vi "DriveDataAQ.vi"(8 "Reset?":bool) -> (2 "Throttle Out":dbl)   [LabVIEW 2015]
uses:
  navX-MXP Library/COMMON/TypeDefs/Data TypeDefs/navX Vector Data.ctl
  navX-MXP Library/navX-MXP IMU.lvlib
panel:
  out "Raw Output Z":dbl[][](array[numeric])
  out "Raw Output Y":dbl[][](array[numeric])
  out "Valid?":bool
  out "Raw Output X":dbl[][](array[numeric])
  out "Linear Acceleration":T1
  in  "Set Throttle":dbl
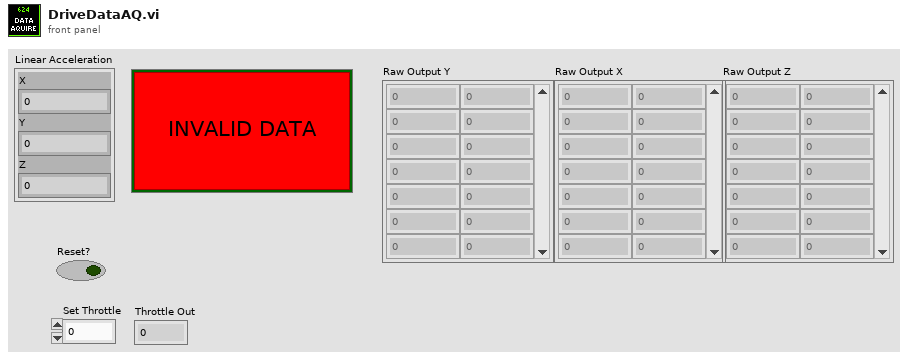
[diagram p1: front panel]
types:
  T1 = typedef "navX-MXP IMU.lvlib/navX Vector Data.ctl" = cluster{"X":dbl, "Y":dbl, "Z":dbl}
  T2 = typedef "navX-MXP IMU.lvlib/navX Device TypeDef.ctl" = cluster{"navX Interface Protocol":T3, "navX Interface Protocol TypeDefs":cluster{"SPIDevRef":T4, "I2CDevRef":T6}, "navX System Information":cluster{"Board Information":T8, "Status":T9, "Offsets":T13}, "navX Common Information":cluster{"Update Rate (4Hz-60Hz)":T14, "refnum name":string, "error":errorcluster}}
  T3 = typedef "navX-MXP IMU.lvlib/navX Interface Protocol.ctl" = enum16{"SPI", "I2C"}
  T4 = typedef "WPI_SPIDevRef.ctl" = cluster{"DevStatus":errorcluster, "Handle":i32, "SPI Bus":T5}
  T5 = typedef "spi_bus.ctl" = enum16{"SPI On-Board, CS0", "SPI On-Board, CS1", "SPI On-Board, CS2", "SPI On-Board, CS3", "SPI MXP", "Invalid"}
  T6 = typedef "WPI_I2CDevRef.ctl" = cluster{"DevStatus":errorcluster, "Device Address":u8, "Handle":i32, "I2C Bus":T7}
  T7 = typedef "i2c_bus.ctl" = enum16{"I2C On-Board", "I2C MXP", "Invalid"}
  T8 = typedef "navX-MXP IMU.lvlib/navX Board Information.ctl" = cluster{"WhoAmI (50 | 0x32)":u8, "Board Revision":u8, "Firmware Major Version":u8, "Firmware Minor Version":u8}
  T9 = typedef "navX-MXP IMU.lvlib/navX Status Data.ctl" = cluster{"Update Rate Hz":u8, "Accelerometer Full-Scale Range":u8, "Gyro Full-Scale Range":u16, "NAVX_OP_STATUS":T10, "NAVX_CAL_STATUS":T11, "NAVX_SELFTEST_STATUS":u8, "NAVX_SENSOR_STATUS":T12}
  T10 = typedef "navX-MXP IMU.lvlib/navX NAVX_OP_STATUS.ctl" = u8
  T11 = typedef "navX-MXP IMU.lvlib/navX NAVX_CAL_STATUS.ctl" = u8
  T12 = typedef "navX-MXP IMU.lvlib/navX NAVX_SENSOR_STATUS.ctl" = cluster{"MOVING":bool, "YAW_STABLE":bool, "MAG_DISTURBANCE":bool, "ALTITUDE_VALID":bool, "SEALEVEL_PRESS_SET":bool, "FUSED_HEADING_VALID":bool}
  T13 = typedef "navX-MXP IMU.lvlib/navX Offsets Data.ctl" = cluster{"Yaw":dbl, "Quat W":dbl, "Quat X":dbl, "Quat Y":dbl, "Quat Z":dbl}
  T14 = typedef "navX-MXP IMU.lvlib/navX Update Rate.ctl" = u8
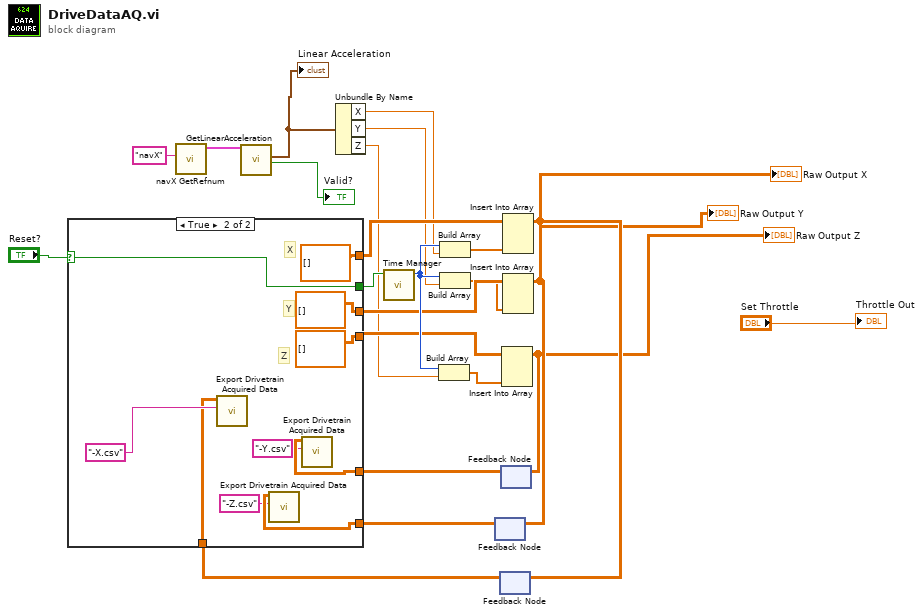
[diagram p0: block diagram]
diagram:
  n1 = call "navX GetRefnum.vi"("refnum name"="navX") -> ("navX Device TypeDef"=w18:T2)  [unwired: 9 in, 1 out]
  n2 = call "GetLinearAcceleration.vi"("navX Device TypeDef"=w18) -> ("Valid?"=→"Valid?":bool, "Linear Acceleration"=w8:T1)  [unwired: 8 in, 1 out]
  "Linear Acceleration" <- w8
  n3 = Unbundle By Name(w8) -> ("X"=w2:dbl, "Y"=w1:dbl, "Z"=w3:dbl)
  n4 = feedback #1() -> (w11:dbl[][])  [unwired: 1 in]
  n5 = feedback #2() -> (w22:dbl[][])  [unwired: 1 in]
  n6 = feedback #3() -> (w10:dbl[][])  [unwired: 1 in]
  n7 = case shown="True" "Reset?" {
    selector: "Reset?" -> [w26 w36]
    tunnel: [w27 dbl[][] []] -> w23
    tunnel: w22 -> [w27 w32]
    tunnel: [w26 w36] -> w20
    tunnel: [w25 dbl[][] []] -> w15
    tunnel: [w24 dbl[][] []] -> w14
    tunnel: w11 -> [w25 w29]
    tunnel: w10 -> [w24 w31]
    frame False {
    }
    frame True {
      # "Z"
      # "Y"
      # "X"
      n8 = call "Export Drivetrain Acquired Data.vi"("string"="-X.csv", "Array"=w32) -> ()  [unwired: 10 in]
      n9 = call "Export Drivetrain Acquired Data.vi"("string"="-Z.csv", "Array"=w29) -> ()  [unwired: 10 in]
      n10 = call "Export Drivetrain Acquired Data.vi"("string"="-Y.csv", "Array"=w31) -> ()  [unwired: 10 in]
    }
  }
  n11 = call "Time Manager.vi"("Reset?"=w20) -> ("Elapsed Time"=w16:u32)  [unwired: 10 in]
  n12 = Build Array(w16, w3) -> (w13:dbl[])
  n13 = Build Array(w16, w2) -> (w19:dbl[])
  n14 = Build Array(w16, w1) -> (w12:dbl[])
  n15 = Insert Into Array(array=w14, new element=w13) -> (w4:dbl[][])  [unwired: 2 in]
  "Raw Output Z" <- w4
  n16 = feedback-in #3(w4) -> ()
  n17 = Insert Into Array(array=w23, new element=w19) -> (w6:dbl[][])  [unwired: 2 in]
  "Raw Output X" <- w6
  n18 = feedback-in #2(w6) -> ()
  n19 = Insert Into Array(array=w15, new element=w12) -> (w5:dbl[][])  [unwired: 2 in]
  "Raw Output Y" <- w5
  n20 = feedback-in #1(w5) -> ()
  "Throttle Out" <- "Set Throttle"
